vi "DisplayConsole.vi"(8 "error in (no error)":errorcluster) -> (0 "error out":errorcluster)   [LabVIEW 2013, in "DisplayConsoleLib.lvlib"]
doc: "Display Console updates the current status of the ATM application"
uses:
  DisplayConsoleLib.lvlib
  PrivateContols/DisplayConsole_QueueDriver.ctl
  Config Database/Private Controls/Queue Driver Control_Config DB.ctl
  UserConsole/PrivateControls/UserConsole_QueueDriver.ctl
  ErrorConsole/PrivateControls/ErrorConsole_QueueDriver.ctl
  UserConsole/UserConsole.lvlib
  MainVI/TopLevelController/ToplevelControllerLibrary.lvlib
  ErrorConsole/ErrorConsoleLib.lvlib
  Config Database/ConfigDBLib.lvlib
panel:
  out "Card Read":bool
  out "Message Screen":string
  out "Current Transaction":string
  # "Display Console updates the current status of the ATM application"
  # "[Covers: UI3]"
  # "[Covers: UI1]"
  # "[Covers: UI3A] \n[Covers: UI3B] \n[Covers: UI3C]"
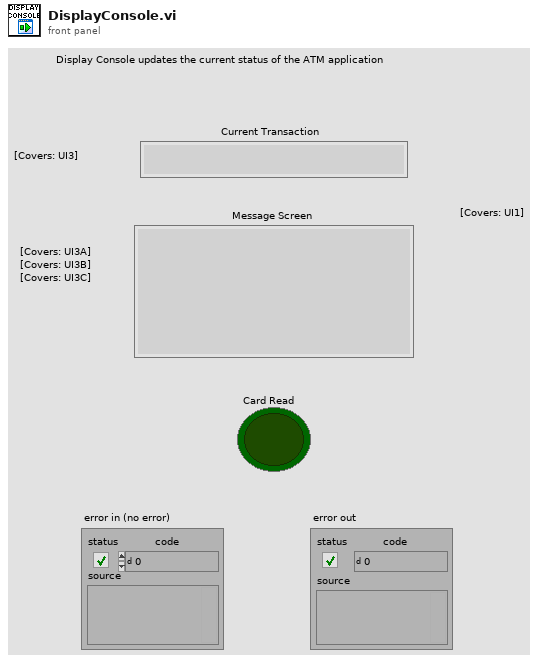
[diagram p1: front panel]
types:
  T1 = typedef "DisplayConsoleLib.lvlib/DisplayConsole_QueueDriver.ctl" = enum16{"Default Case", "Init", "Enqueue", "Dequeue", "ReleaseQueue", "Exit"}
  T2 = enum16{"Create Event", "Generate Event", "Destroy Event"}
  T3 = typedef "ConfigDBLib.lvlib/Queue Driver Control_Config DB.ctl" = enum16{"Init", "Enqueue", "Dequeue", "ReleaseQueue", "Exit"}
  T4 = typedef "UserConsole.lvlib/UserConsole_QueueDriver.ctl" = enum16{"Default Case", "Init", "Enqueue", "Dequeue", "ReleaseQueue", "Exit"}
  T5 = enum16{"Init", "Enqueue", "Dequeue", "ReleaseQueue", "Exit"}
  T6 = typedef "ErrorConsoleLib.lvlib/ErrorConsole_QueueDriver.ctl" = enum16{"Default", "Init", "Enqueue", "Dequeue", "ReleaseQueue", "Exit"}
  T7 = cluster{"Current Transaction":string, "Message Screen":string, "Card Read":bool}
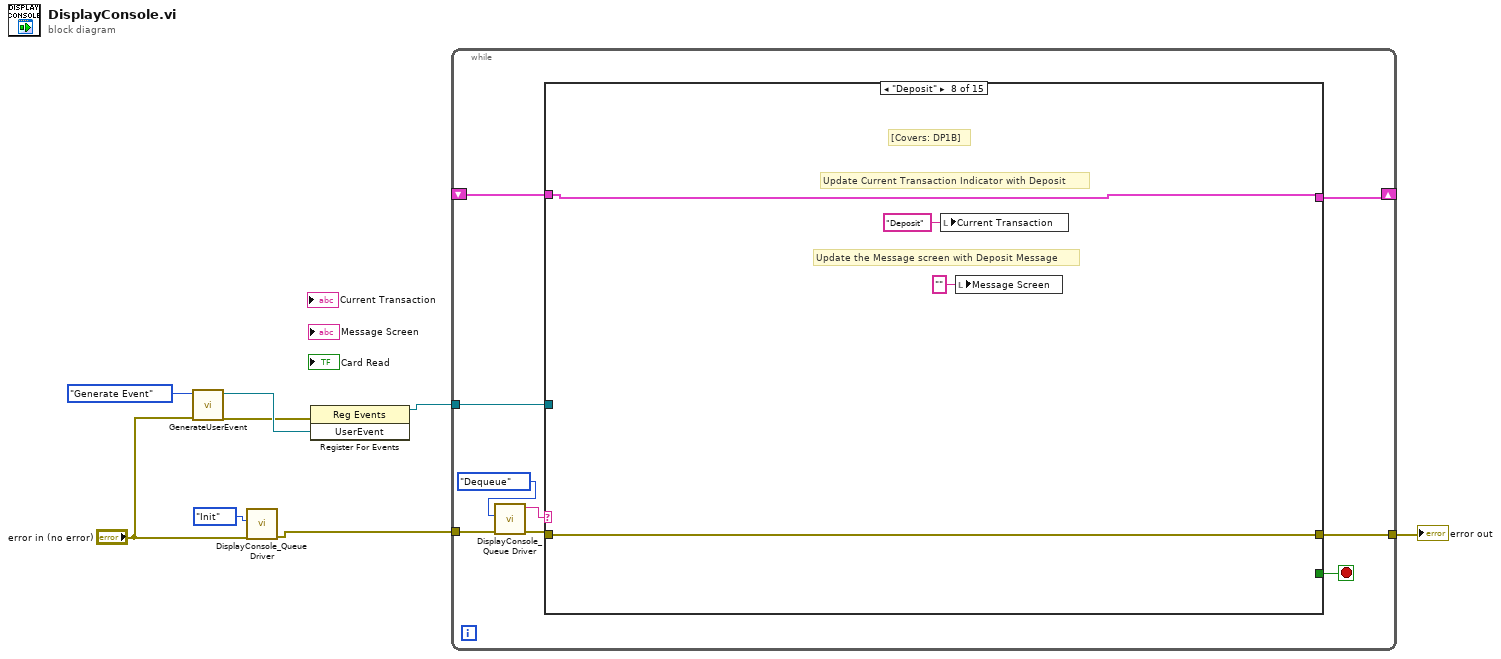
[diagram p0: block diagram]
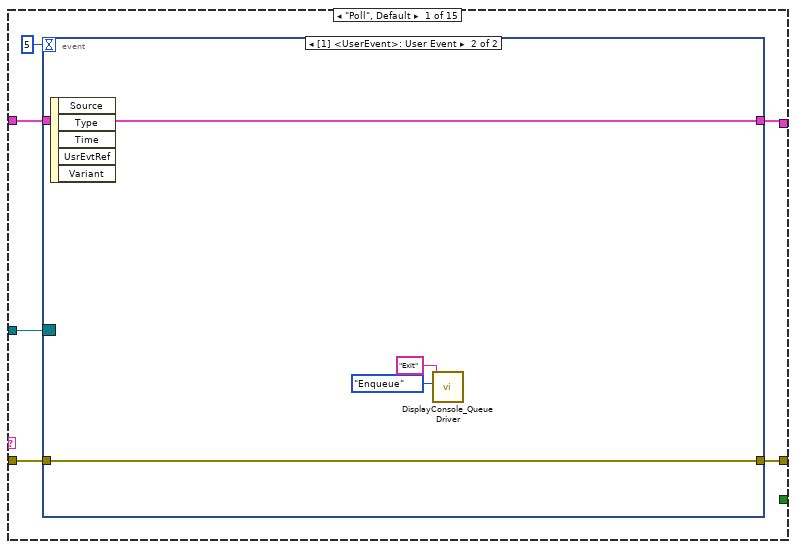
[diagram p2: hidden frame]
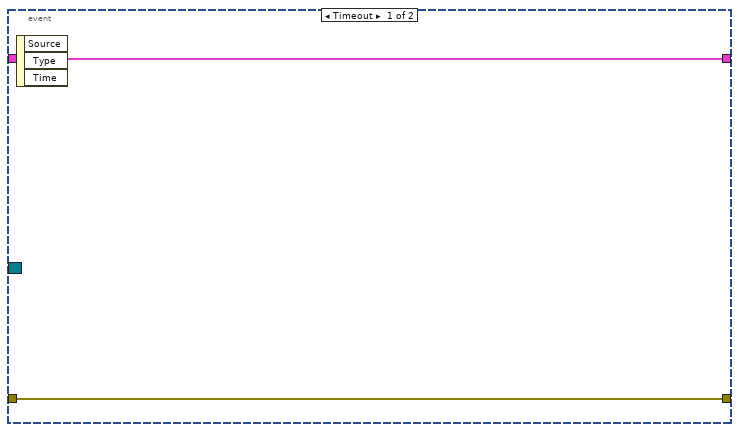
[diagram p3: hidden frame]
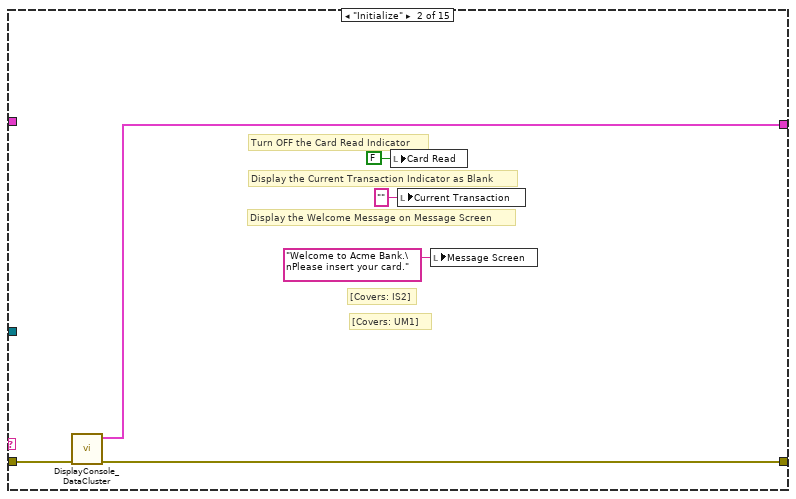
[diagram p4: hidden frame]
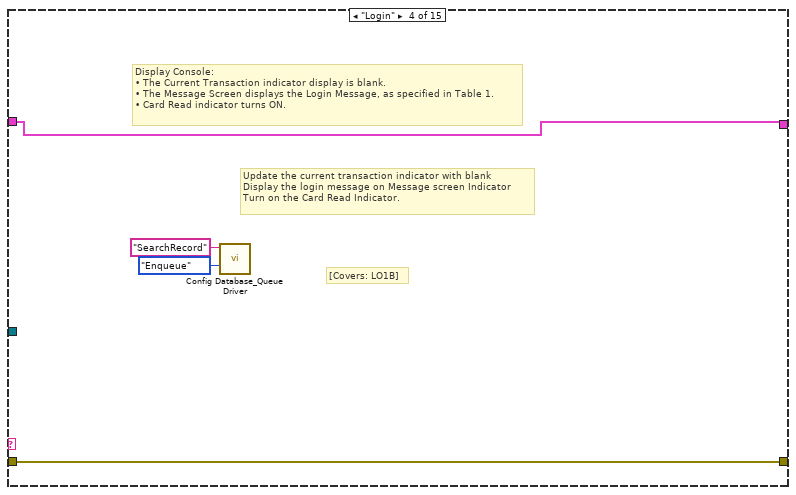
[diagram p6: hidden frame]
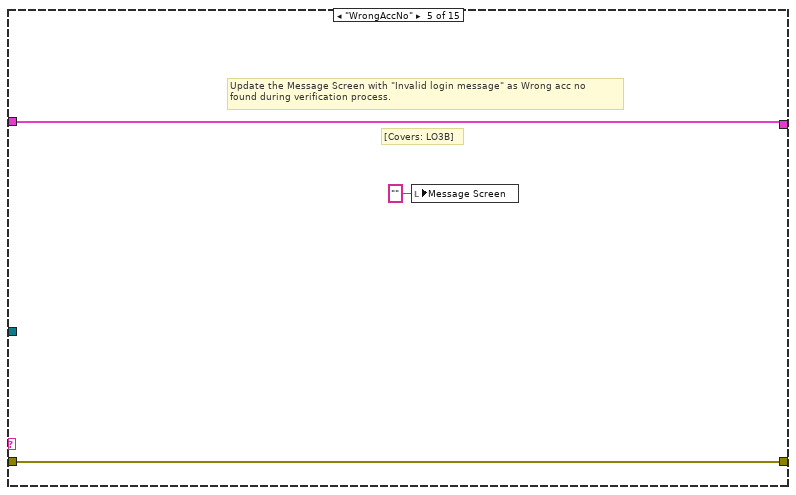
[diagram p7: hidden frame]
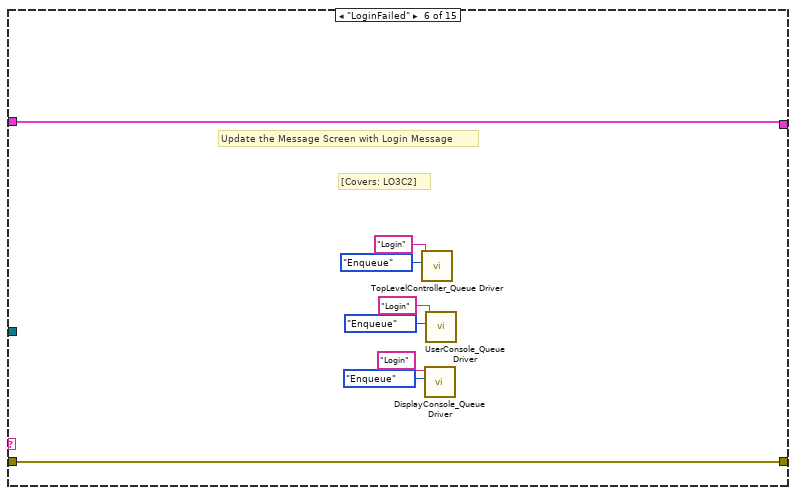
[diagram p8: hidden frame]
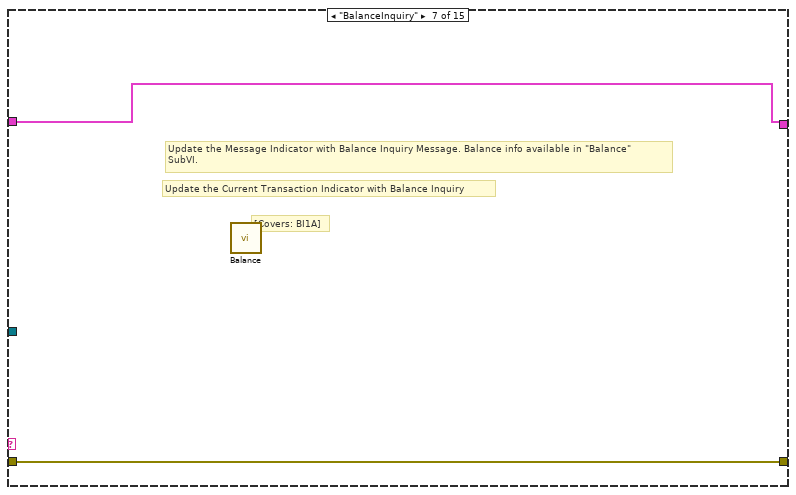
[diagram p9: hidden frame]
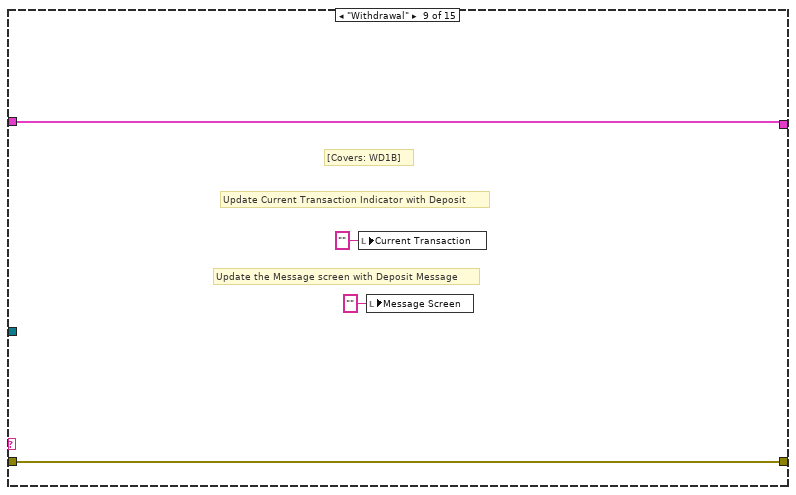
[diagram p10: hidden frame]
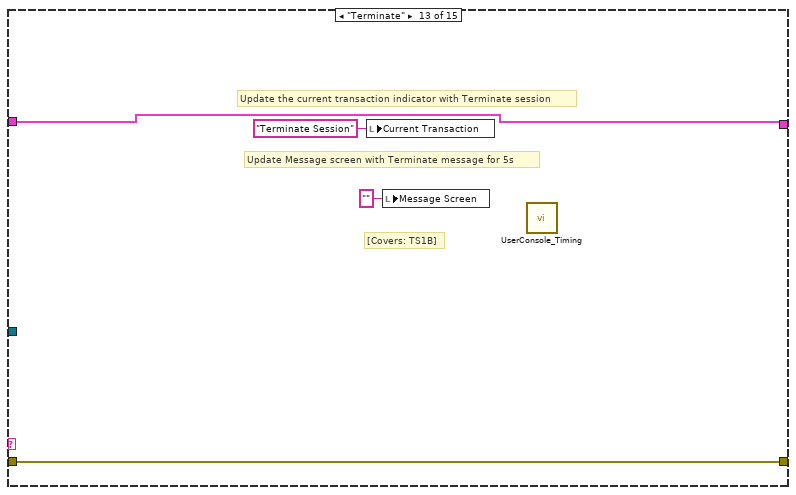
[diagram p14: hidden frame]
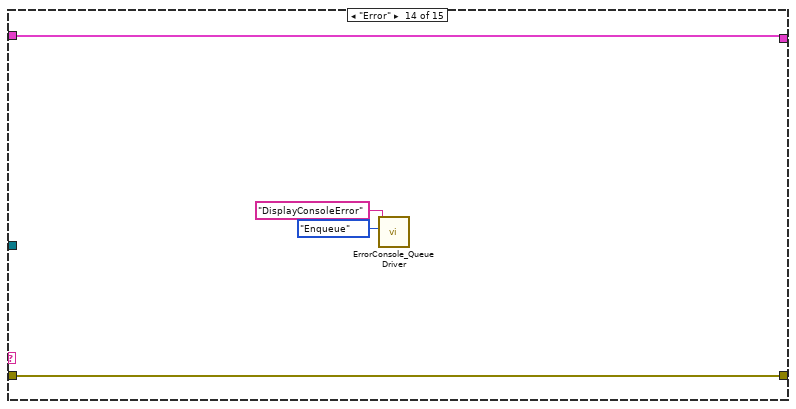
[diagram p15: hidden frame]
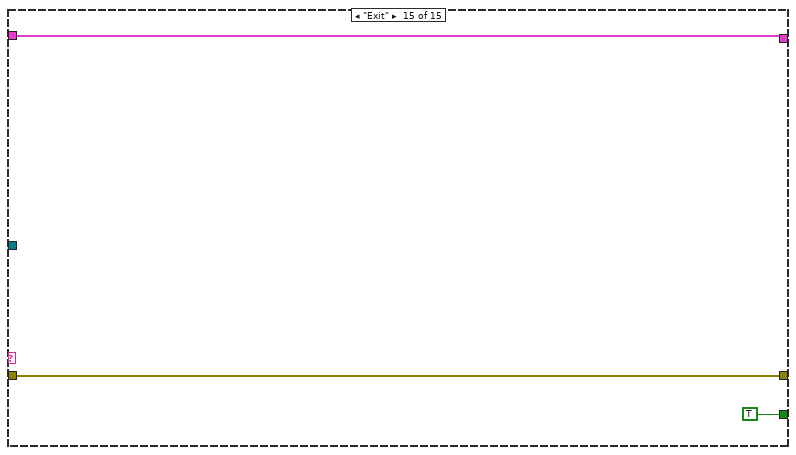
[diagram p16: hidden frame]
diagram:
  n1 = call "GenerateUserEvent.vi"("error in (no error)"="error in (no error)", "Event Actions"=T2."Generate Event") -> ("error out"=w4:errorcluster, "UserEvent"=w5:refnum<user-event>)  [unwired: 8 in]
  n2 = call "DisplayConsole_Queue Driver.vi"("error in (no error)"="error in (no error)", "State"=DisplayConsole_QueueDriver."Init") -> ("error out"=w7:errorcluster)  [unwired: 8 in, 1 out]
  n3 = register-events(error in=w4, w5) -> (reference out=w3:refnum<event-registration>)  [unwired: 1 in, 1 out]
  n4 = while {
    tunnel: [w17] -> w8
    shift-right: [w16] -> _
    shift-left: _ -> [w15]
    tunnel: w7 -> [w13]
    tunnel: w3 -> [w10]
    stop <- w14 stop-if-true
    n5 = call "DisplayConsole_Queue Driver.vi"("error in (no error)"=w13, "State"=DisplayConsole_QueueDriver."Dequeue") -> ("error out"=w12:errorcluster, "DeQ"=w11:string)  [unwired: 8 in]
    n6 = case shown="\"Deposit\"" w11 {
      tunnel: [w19 w34 w37 w41 w43 w52 w54 w56 w62 w64 w66 w68 w69 w76 w79] -> w17
      tunnel: w12 -> [w20 w35 w37 w41 w43 w52 w54 w56 w62 w64 w66 w68 w69 w76 w79]
      tunnel: [w21 w33 w36 w40 w44 w51 w53 w55 w61 w63 w65 w67 w70 w75 w78] -> w16
      tunnel: w15 -> [w22 _ w36 w40 w44 w51 w53 w55 w61 w63 w65 w67 w70 w75 w78]
      tunnel: [_ _ _ _ _ _ _ _ _ _ _ _ _ _ TRUE] -> w14
      tunnel: w10 -> [w18 _ _ _ _ _ _ _ _ _ _ _ _ _ _]
      frame "Poll", Default {
        n7 = event shown="[1] <UserEvent>: User Event" {
          selector: w18 -> [_ _]
          dyn-events: _ -> [_ _]
          timeout: 5 -> [_ _]
          tunnel: w22 -> [w25 w27]
          tunnel: [w25 w27] -> w21
          tunnel: w20 -> [w24 w29]
          tunnel: [w24 w29] -> w19
          event Timeout {
            n8 = event-data() -> ()  [unwired: 1 in, 3 out]
          }
          event User Event {
            n9 = event-data() -> ()  [unwired: 1 in, 5 out]
            n10 = call "DisplayConsole_Queue Driver.vi"("State"=DisplayConsole_QueueDriver."Enqueue", "EnQ"="Exit") -> ()  [unwired: 8 in, 2 out]
          }
        }
      }
      frame "Initialize" {
        # "[Covers: UM1]"
        # "[Covers: IS2]"
        # "Display the Welcome Message on Message Screen"
        # "Display the Current Transaction Indicator as Blank"
        # "Turn OFF the Card Read Indicator"
        n11 = call "DisplayConsole_DataCluster.vi"("error in (no error)"=w35) -> ("error out"=w34:errorcluster, "DataCluster"=w33:T7)  [unwired: 9 in]
        n12 = local write "Card Read"(FALSE ("Card Read")) -> ()
        n13 = local write "Current Transaction"("" ("Current Transaction")) -> ()
        n14 = local write "Message Screen"("Welcome to Acme Bank.\nPlease insert your card." ("Message Screen")) -> ()
      }
      frame "Idle" {
        # "[Covers: ID1B]"
        # "Display the Idle message on Message Indicator"
        # "Display the New Transaction on Current Transaction Indicator"
      }
      frame "Login" {
        # "[Covers: LO1B]"
        # "Update the current transaction indicator with blank\nDisplay the login message on Message screen Indicator\nTurn on the Card Read Indicator."
        # "Display Console:\n• The Current Transaction indicator display is blank.\n• The Message Screen displays the Login Message, as specified in Table 1.\n• Card Read indicator turns ON."
        n15 = call "Config Database_Queue Driver.vi"("Enum"=Queue_Driver_Control_Config_DB."Enqueue", "EnQ"="SearchRecord") -> ()  [unwired: 8 in, 2 out]
      }
      frame "WrongAccNo" {
        # "[Covers: LO3B]"
        # "Update the Message Screen with \"Invalid login message\" as Wrong acc no \nfound during verification process."
        n16 = local write "Message Screen"("" ("Message Screen")) -> ()
      }
      frame "LoginFailed" {
        # "[Covers: LO3C2]"
        # "Update the Message Screen with Login Message"
        n17 = call "TopLevelController_Queue Driver.vi"("Enum"=T5."Enqueue", "EnQ"="Login") -> ()  [unwired: 8 in, 2 out]
        n18 = call "DisplayConsole_Queue Driver.vi"("State"=DisplayConsole_QueueDriver."Enqueue", "EnQ"="Login") -> ()  [unwired: 8 in, 2 out]
        n19 = call "UserConsole_Queue Driver.vi"("State"=UserConsole_QueueDriver."Enqueue", "EnQ"="Login") -> ()  [unwired: 8 in, 2 out]
      }
      frame "BalanceInquiry" {
        # "[Covers: BI1A]"
        # "Update the Current Transaction Indicator with Balance Inquiry"
        # "Update the Message Indicator with Balance Inquiry Message. Balance info available in \"Balance\"\nSubVI."
        n20 = call "Balance.vi"() -> ()  [unwired: 12 in]
      }
      frame "Deposit" {
        # "[Covers: DP1B]"
        # "Update Current Transaction Indicator with Deposit"
        # "Update the Message screen with Deposit Message"
        n21 = local write "Current Transaction"("Deposit" ("Current Transaction")) -> ()
        n22 = local write "Message Screen"("" ("Message Screen")) -> ()
      }
      frame "Withdrawal" {
        # "Update Current Transaction Indicator with Deposit"
        # "Update the Message screen with Deposit Message"
        # "[Covers: WD1B]"
        n23 = local write "Current Transaction"("" ("Current Transaction")) -> ()
        n24 = local write "Message Screen"("" ("Message Screen")) -> ()
      }
      frame "WithdrawalComplete" {
        # "If suffiecient fund availble, Update the Withdrawalcomplete message on Message\nscreen"
        # "[Covers: WD1D]"
      }
      frame "WithdrawalFailed" {
        # "If suffiecient Fund unavailble, Update the WithdrawalFailed message on Message\nscreen"
        # "[Covers: WD1E]"
      }
      frame "Fast Cash $50" {
        # "[Covers: FC1B]"
        # "Update Current Transaction Indicator with Fast Cash $50"
        # "Update the Message screen with Fast Cash $50 Message"
      }
      frame "Terminate" {
        # "[Covers: TS1B]"
        # "Update Message screen with Terminate message for 5s"
        # "Update the current transaction indicator with Terminate session"
        n25 = local write "Current Transaction"("Terminate Session" ("Current Transaction")) -> ()
        n26 = local write "Message Screen"("" ("Message Screen")) -> ()
        n27 = call "UserConsole_Timing.vi"() -> ()  [unwired: 11 in, 1 out]
      }
      frame "Error" {
        n28 = call "ErrorConsole_Queue Driver.vi"("State"=ErrorConsole_QueueDriver."Enqueue", "EnQ"="DisplayConsoleError") -> ()  [unwired: 8 in, 2 out]
      }
      frame "Exit" {
      }
    }
  }
  "error out" <- w8
